vi "executeDefendAreaSkill.vi"(6 "Number of Defenders\nWithout Duelist":i32, 8 "error in (no error)":errorcluster, 9 "Robot in":refnum<class "Robot.lvclass">, 10 "Game":refnum<class "Game.lvclass">, 11 "DefendAreaSkill in":refnum<class "DefendAreaSkill.lvclass">) -> (0 "error out":errorcluster, 2 "Robot out":refnum<class "Robot.lvclass">, 3 "DefendAreaSkill out":refnum<class "DefendAreaSkill.lvclass">)   [LabVIEW 2024, in "DefendAreaSkill.lvclass"]
uses:
  DefendAreaSkill.lvclass
  Game_class/Game.lvclass
  Robot_class/Robot.lvclass
  Utilities_class/Utilities.lvclass
  Team_class/DefensivePlay.ctl
  Team_class/OffensivePlay.ctl
  Game_class/Game.lvclass/Game.ctl
  Parameters_class/Parameters.lvclass/Parameters.ctl
  Team_class/Team.lvclass/Team.ctl
  Robot_class/Robot.lvclass/Robot.ctl
  Game_class/Read Utilities.lvclass.vi
  Game_class/Read FieldRef.vi
  Game_class/Read BallRef.vi
  Robot_class/Write kick_x.vi
  Robot_class/Write kick_z.vi
  Game_class/Read NewParameters.vi
  Game_class/Read OffensiveTeam.vi
  Team_class/Read OffensivePlay.vi
  Game_class/Read Parameters.lvclass.vi
  Game_class/Read DefensiveTeam.vi
  Team_class/Read RobotRef.vi
  Team_class/Read DefensivePlay.vi
  Parameters_class/Read minDistanceToPass.vi
  Parameters_class/Read Enviroment.vi
  Parameters_class/Read MinDistToKick.vi
  Parameters_class/Read ChipKick activated.vi
  Parameters_class/Read ChipKick Force 1.vi
  Parameters_class/Read KickForce.vi
  Parameters_class/Read PassForceMult.vi
  Parameters_class/Read Area.vi
  Robot_class/Write dest_x.vi
  Robot_class/Write dest_y.vi
  Robot_class/Write dest_orientation.vi
  Robot_class/Read orientation.vi
  Ally_class/Ally.lvclass
  C:/Users/ROBOIME2/Documents/SSL ROBOIME/SSL_AI/Team_class/Team.lvclass
  Ball_class/Ball.lvclass
  Parameters_class/Parameters.lvclass
  Field_class/Field.lvclass
  KickToSkill_class/KickToSkill.lvclass
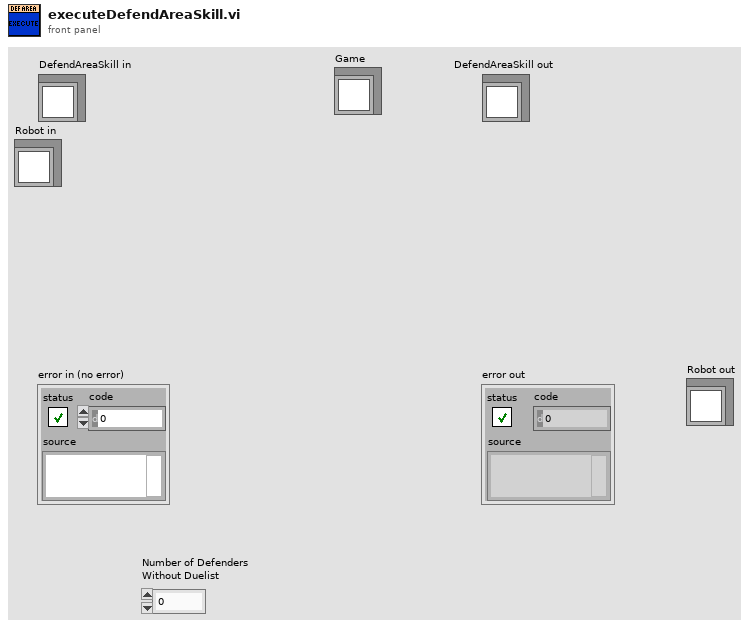
[diagram p1: front panel]
types:
  T1 = typedef "OffensivePlay.ctl" = enum16{"5RobotsPassGamePlay", "5PreparePassGame", "5RobotsKeeperGame", "KeeperPassToStriker", "5RobotsNormalGamePlay", "PrepareKeeperPass", "ACBPass", "ABCPass", "PrepareTriplePass", "TableWithStriker", "TableWith2ndStrikerPlay", "PrepareDoublePass", "PrepareRollToPass", "SimplePass", "PreparePass", "PassToStriker", "BallOutOfField", "PassTo2ndStriker", "StopOffensive", "Prepare Penalty Enemy", "EnemyPossessionAtEnemyField", "EnemyPossesionAtOurField", "TestPlay", "PreparePenaltyAlly", "KickPenaltyAlly", "PrepareKickoffAlly", "PrepareKickoffEnemy", "IndirectEnemy", "DirectEnemy", "PreparePassInGame1", "NormalGame", "DirectKick", "Pass", "Halt", "Timeout", "PassPlay", "PenaltyEnemy"}
  T2 = typedef "DefensivePlay.ctl" = enum16{"NormalDefensiveWithDuelist", "NormalDefensive", "TestPlay", "Halt", "Timeout", "PenaltyEnemy", "PenaltyAlly", "StopDefensive"}
  T3 = typedef "Enviroment.ctl" = enum16{"erForceSimulator", "grSim", "realGame"}
  T4 = typedef "NewParameters.ctl" = cluster{"PenaltyDistance":dbl, "DistanceAttackerToBackBall":dbl, "Division":enum16{"Div B", "Div A"}, "DistanceToAvoidyEnemyRobot":dbl, "BallPlacementDistance":dbl, "DisatanceBehindBallToStealBall":dbl, "MaxDistanceToPositionKickoff":dbl, "BlockEnemyTarget":bool, "MaxStopVAng":dbl, "DistanceMarkerToEnemy":dbl, "IgnoreDribblerContact":bool, "DistanceToBeginEnemyPosession":dbl, "GoToBallWhenEnemyNotMoving":bool, "EnemyDistanceToReduceVelocity":dbl, "TurnOnEnemyDistanceToReduceVelocity":bool, "EnemyDistanceToShootOutBall":dbl, "DefenseKickBall":bool, "MoreKickToGoal? (0-0.3)":dbl, "ChipKickInEnemyField":bool, "ShootOutRobotId":dbl, "FieldLenghtDenominatorInShootOut":dbl, "AdjustPositionInBallPlacement":bool, "PowerGodPass":dbl, "VelocityAbortEnemyPos":dbl, "MaxDistToBeginPass":dbl, "MinDistToBeginPass":dbl, "VelocityInDirects":dbl, "BadDribblerIDs":i32[], "NewKickToDistanceAroundBall":dbl, "PowerAvoidColisionMarker":dbl, "DistanceToAvoidColisionMarker":dbl, "AvoidBallKick":dbl, "DistanceTryKick":dbl, "SuicideKickDIstance":dbl, "AdjustFirstKickDistance":dbl, "AvoidAimLessKick":dbl, "DistanceToAvoidyEnemyShootRobot ":dbl, "NumberOfMarkers":dbl, "PotField":bool, "PIDLateral":bool, "MinDistanceFirstKickX":dbl, "MinDistanceFirstKickY":dbl, "FractionOfDistToTouchGround\nAfterChipKick":dbl, "FractionOfKickxWhen\nComposedWithKickz":dbl, "Style":T5, "MoveInTurnState":bool, "DistFromEnemyToConsider\nMoveInTurnState":dbl, "CascadePID":bool, "TurnAroundParameters":cluster{"Radius":dbl, "Multiplier":dbl, "ChordAngle":dbl}, "SafeDriveVel":dbl, "DistanceToGoToBackBall":dbl, "minDistanceToNotFinish\nEnemyPossession":dbl, "OneTouchShot":cluster{"angleFactor":dbl, "maxAngle":dbl, "Attack":bool, "Defense":bool}, "OpenAngleToGoal":cluster{"minAngle":dbl, "maxAngle":dbl, "minEvaluation":dbl}, "ShotInterception":cluster{"shotSpeed":dbl, "minEnemySpeed":dbl, "maxEnemySpeed":dbl, "minEvaluation":dbl}, "AllyTeamArray":T6[], "maxDefendersNumber":i32, "Zone":cluster{"GuardPositionArray":dbl[][], "ZoneMidField":dbl[], "CenterForwardWidth":dbl}, "MinEvaluationToShoot":dbl, "PassInterception":cluster{"maxPassSpeed":dbl, "minPassSpeed":dbl, "minEnemySpeed":dbl, "chipPassDistance":dbl, "chipPassEvaluation":dbl, "minEvaluation":dbl, "maxEnemySpeed":dbl}, "PassDistance":cluster{"maxDistance":dbl, "minDistance":dbl}, "receiverSpeed":dbl, "maxBallSpeed":dbl, "slackTime":dbl, "Turning radius":dbl, "Turning v_ang":dbl, "AlignError":cluster{"Distance":dbl, "Orientation":dbl, "V_norm(m/s)":dbl, "V_ang (rad/s)":dbl}, "RobotRadius":dbl, "KickerDistance":dbl, "keeper angle  to cover goalpost":dbl, "a_slide":dbl, "a_roll":dbl, "k_switch":dbl}
  T5 = typedef "Style.ctl" = enum16{"Insanity", "Offensive", "Defensive"}
  T6 = typedef "AllyTeam.ctl" = enum16{"Keeper", "Defender", "Attacker"}
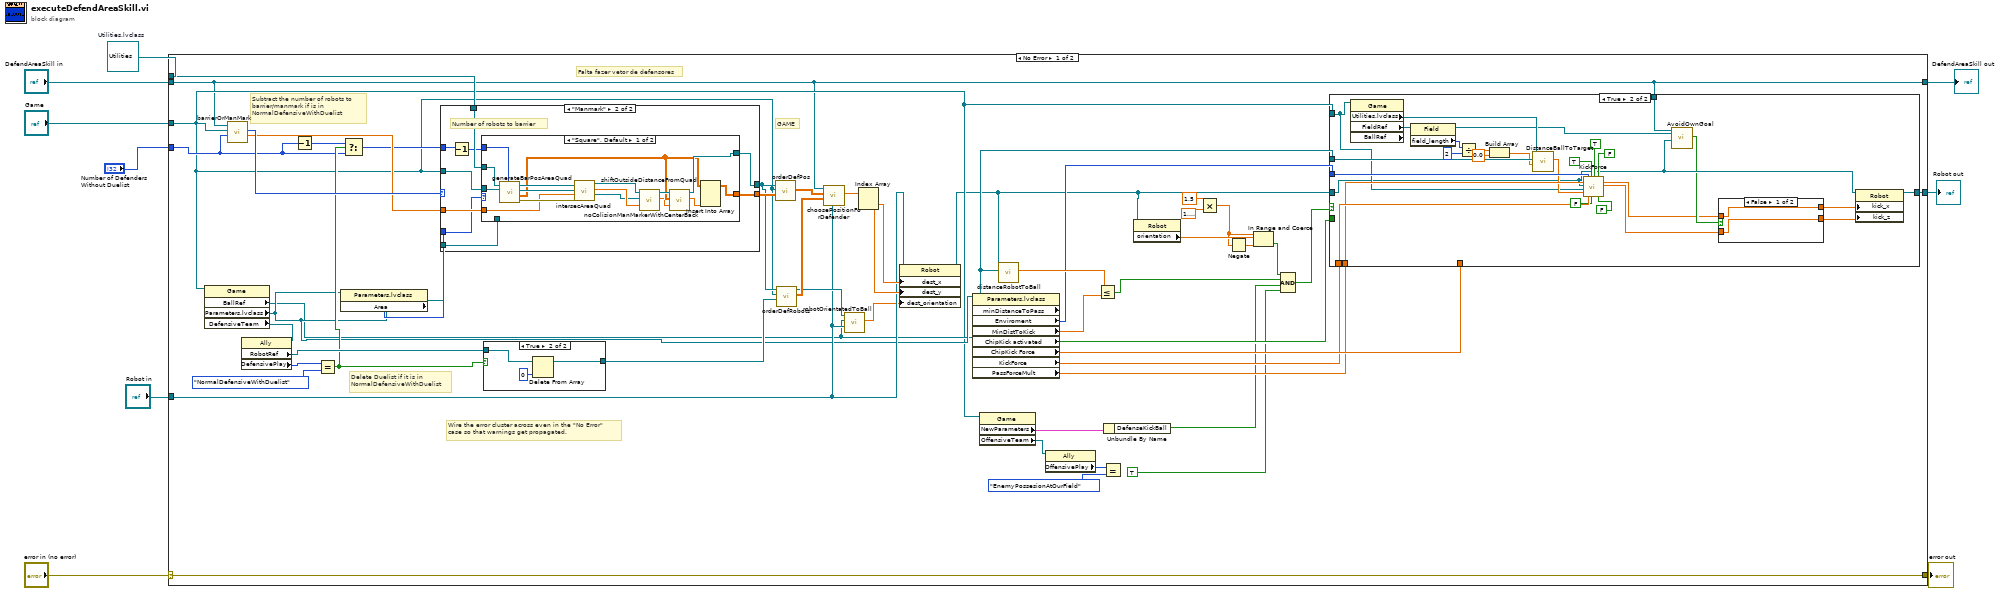
[diagram p0: block diagram]
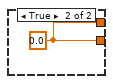
[diagram p3: hidden frame]
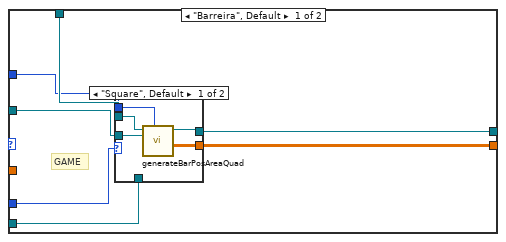
[diagram p5: hidden frame]
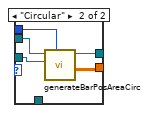
[diagram p6: hidden frame]
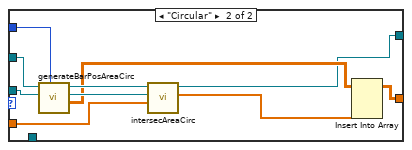
[diagram p7: hidden frame]
diagram:
  w4 = refnum<class "Utilities.lvclass"> refnum  # Utilities.lvclass
  n1 = case shown="No Error" "error in (no error)" {
    selector: "error in (no error)" -> [w60 w150]
    tunnel: [w60 w150] -> w8
    tunnel: [w10 w149] -> w6
    tunnel: "DefendAreaSkill in" -> [w10 w149]
    tunnel: "Game" -> [w24 _]
    tunnel: w4 -> [w58 _]
    tunnel: "Robot in" -> [w48 w148]
    tunnel: [w33 w148] -> w2
    tunnel: "Number of Defenders\nWithout Duelist" -> [w37 _]
    frame No Error {
      # "GAME"
      # "Subtract the number of robots to\nbarrier/manmark if is in\nNormalDefensiveWithDuelist"
      # "Delete Duelist if it is in\nNormalDefensiveWithDuelist"
      # "Falta fazer vetor de defensores"
      # "Wire the error cluster across even in the \"No Error\"\ncase so that warnings get propagated."
      n2 = property class="Game"(reference=w24) -> ("BallRef"=w27:refnum<class "Ball.lvclass">, "Parameters.lvclass"=w35:refnum<class "Parameters.lvclass">, "DefensiveTeam"=w45:refnum<class "Ally.lvclass">)  [unwired: 1 in, 2 out]
      n3 = call "barrierOrManMark.vi"("Number of Defenders\nWithout Duelist"=w37, "Game"=w24, "DefendAreaSkill in"=w10) -> ("Enemy position\nto mark"=w55:dbl[], "Type of Defense Barrier"=w59:enum16{"Barreira", "Manmark"})  [unwired: 5 in, 2 out]
      n4 = property class="Ally"(reference=w45) -> ("RobotRef"=w41:refnum<class "Robot.lvclass">[], "DefensivePlay"=w44:T2)  [unwired: 1 in, 2 out]
      n5 = Decrement(x=w37) -> (x-1=w39:i32)
      n6 = Equal?(x=w44, y=DefensivePlay."NormalDefensiveWithDuelist") -> (x = y?=w40:bool)
      n7 = property class="Parameters.lvclass"(reference=w35) -> ("Area"=w46:enum16{"Circular", "Square"})  [unwired: 1 in, 2 out]
      n8 = Select(t=w39, s=w40, f=w37) -> (s? t:f=w38:i32)
      n9 = case shown="\"Manmark\"" w59 {
        tunnel: w46 -> [w102 w115]
        tunnel: w58 -> [w101 w119]
        tunnel: w35 -> [w100 w121]
        tunnel: w24 -> [w99 w120]
        tunnel: [w98 w117] -> w57
        tunnel: [w97 w116] -> w56
        tunnel: w55 -> [_ w118]
        tunnel: w38 -> [w96 w114]
        frame "Barreira", Default {
          # "GAME"
          n10 = case shown="\"Square\", Default" w102 {
            tunnel: w101 -> [w107 w112]
            tunnel: w100 -> [_ _]
            tunnel: w99 -> [w106 w111]
            tunnel: [w105 w110] -> w97
            tunnel: [w104 w109] -> w98
            tunnel: w96 -> [w103 w108]
            frame "Square", Default {
              n11 = call "generateBarPosAreaQuad.vi"("Number of Defenders\nWithout Duelist"=w103, "Game"=w106, "Utilities in"=w107) -> ("Pos Centers Back"=w104:dbl[][], "Utilities out"=w105:refnum<class "Utilities.lvclass">)  [unwired: 5 in, 2 out]
            }
            frame "Circular" {
              n12 = call "generateBarPosAreaCirc.vi"("Number of Denfenders\nWhithout Duelist"=w108, "Game"=w111, "Utilities in"=w112) -> ("Posição dos Defensores"=w109:dbl[][], "Utilities out"=w110:refnum<class "Utilities.lvclass">)  [unwired: 5 in, 2 out]
            }
          }
        }
        frame "Manmark" {
          # "Number of robots to barrier"
          n13 = Decrement(x=w114) -> (x-1=w113:i32)
          n14 = case shown="\"Square\", Default" w115 {
            tunnel: w119 -> [w137 w147]
            tunnel: w121 -> [_ _]
            tunnel: w120 -> [w136 w146]
            tunnel: w118 -> [w132 w143]
            tunnel: [w131 w140] -> w117
            tunnel: [w125 w139] -> w116
            tunnel: w113 -> [w130 w138]
            frame "Square", Default {
              n15 = call "generateBarPosAreaQuad.vi"("Number of Defenders\nWithout Duelist"=w130, "Game"=w136, "Utilities in"=w137) -> ("error out"=w135:errorcluster, "Pos Centers Back"=w124:dbl[][], "Game out"=w133:refnum<class "Game.lvclass">, "Utilities out"=w134:refnum<class "Utilities.lvclass">)  [unwired: 5 in]
              n16 = call "intersecAreaQuad.vi"("error in (no error)"=w135, "Ball/Enemy\nPosition"=w132, "Game"=w133, "Utilities in"=w134) -> ("Game"=w127:refnum<class "Game.lvclass">, "Pos de Interseção"=w129:dbl[], "Utilities out"=w128:refnum<class "Utilities.lvclass">)  [unwired: 4 in, 1 out]
              n17 = call "shiftOutsideDistanceFromQuad.vi"("Pos de Interseção"=w129, "Game"=w127, "Utilities in"=w128) -> ("Array"=w123:dbl[], "Utilities out"=w126:refnum<class "Utilities.lvclass">)  [unwired: 6 in, 1 out]
              n18 = call "noColisionManMarkerWithCenterBack.vi"("Pos ManMarker 2"=w123, "Pos CenterBacks"=w124, "Utilities in"=w126) -> ("Pos ManMarker"=w122:dbl[], "Utilities out"=w125:refnum<class "Utilities.lvclass">)  [unwired: 6 in, 1 out]
              n19 = Insert Into Array(array=w124, new element=w122) -> (w131:dbl[][])  [unwired: 2 in]
            }
            frame "Circular" {
              n20 = call "generateBarPosAreaCirc.vi"("Number of Denfenders\nWhithout Duelist"=w138, "Game"=w146, "Utilities in"=w147) -> ("Posição dos Defensores"=w142:dbl[][], "Game out"=w144:refnum<class "Game.lvclass">, "Utilities out"=w145:refnum<class "Utilities.lvclass">)  [unwired: 5 in, 1 out]
              n21 = call "intersecAreaCirc.vi"("Ball/Enemy\nPosition"=w143, "Game"=w144, "Utilities in"=w145) -> ("Position"=w141:dbl[], "Utilities out"=w139:refnum<class "Utilities.lvclass">)  [unwired: 6 in, 1 out]
              n22 = Insert Into Array(array=w142, new element=w141) -> (w140:dbl[][])  [unwired: 2 in]
            }
          }
        }
      }
      n23 = case shown="True" w40 {
        tunnel: [w92 w95] -> w42
        tunnel: w41 -> [w92 w94]
        frame False {
        }
        frame True {
          n24 = Delete From Array(array=w94, index=0) -> (array with subset deleted=w95:refnum<class "Robot.lvclass">[])  [unwired: 1 in, 1 out]
        }
      }
      n25 = call "orderDefPos.vi"("Def Positions"=w57, "Game"=w24, "Utilities in"=w56) -> ("Ordered Positions"=w54:dbl[][])  [unwired: 6 in, 2 out]
      n26 = call "orderDefRobots.vi"("Array of Robots"=w42, "Game"=w24, "Utilities in"=w56) -> ("Odered array of robots"=w53:dbl[][], "Utilities out"=w49:refnum<class "Utilities.lvclass">)  [unwired: 6 in, 1 out]
      n27 = call "choosePositionForDefender.vi"("Robot"=w48, "Odered array of robots"=w53, "Ordered Positions To Go"=w54, "DefendAreaSkill in"=w10) -> ("Position"=w52:dbl[])  [unwired: 5 in, 2 out]
      n28 = call "robotOrientatedToBall.vi"("Robot"=w48, "BallRef"=w27, "Utilities in"=w49) -> ("Orientation"=w47:dbl)  [unwired: 6 in, 2 out]
      n29 = Index Array(array=w52) -> (element #1=w51:dbl, element #2=w50:dbl)  [unwired: 2 in]
      n30 = property class="Robot"(reference=w48, "dest_x"=w51, "dest_y"=w50, "dest_orientation"=w47) -> (reference out=w18:refnum<class "Robot.lvclass">)  [unwired: 1 in, 1 out]
      n31 = property class="Parameters.lvclass" props=["minDistanceToPass", "Enviroment", "MinDistToKick", "ChipKick activated", "ChipKick Force", "KickForce", "PassForceMult"](reference=w35) -> ("Enviroment"=w30:T3, "MinDistToKick"=w34:dbl, "ChipKick activated"=w32:bool, "ChipKick Force"=w31:dbl, "KickForce"=w29:dbl, "PassForceMult"=w28:dbl)  [unwired: 1 in, 3 out]
      n32 = property class="Game"(reference=w24) -> ("NewParameters"=w23:T4, "OffensiveTeam"=w21:refnum<class "Ally.lvclass">)  [unwired: 1 in, 2 out]
      n33 = call "distanceRobotToBall.vi"("Robot"=w18, "Ball"=w27) -> ("Distance Robot To Ball"=w36:dbl)  [unwired: 7 in, 2 out]
      n34 = property class="Ally"(reference=w21) -> ("OffensivePlay"=w20:T1)  [unwired: 1 in, 2 out]
      n35 = Less Or Equal?(x=w36, y=w34) -> (x <= y?=w25:bool)
      n36 = Equal?(x=w20, y=OffensivePlay."EnemyPossesionAtOurField") -> ()  [unwired: 1 out]
      n37 = Unbundle By Name(w23) -> ("DefenseKickBall"=w22:bool)
      n38 = property class="Robot"(reference=w18) -> ("orientation"=w17:dbl)  [unwired: 1 in, 2 out]
      n39 = Multiply(x=1.5, y=1.5707963267948966) -> (x*y=w12:dbl)
      n40 = Negate(x=w12) -> (-x=w16:dbl)
      n41 = In Range and Coerce(upper limit=w12, x=w17, lower limit=w16) -> (In Range?=w15:bool)  [unwired: 1 out]
      n42 = Compound Arithmetic op=AND(w15, w25, w22, TRUE ("value")) -> (w26:bool)
      n43 = case shown="True" w26 {
        tunnel: w18 -> [w61 w67]
        tunnel: [w61 w88] -> w33
        tunnel: w32 -> [_ _]
        tunnel: w31 -> [_ _]
        tunnel: w30 -> [_ w87]
        tunnel: w29 -> [_ w85]
        tunnel: w28 -> [_ w84]
        tunnel: w27 -> [_ w83]
        tunnel: w24 -> [_ w73]
        tunnel: w10 -> [_ w69]
        frame False {
        }
        frame True {
          n44 = property class="Game" props=["Utilities.lvclass", "FieldRef", "BallRef"](reference=w73) -> ("Utilities.lvclass"=w75:refnum<class "Utilities.lvclass">, "FieldRef"=w81:refnum<class "Field.lvclass">)  [unwired: 1 in, 3 out]
          n45 = property class="Field"(reference=w81) -> (reference out=w68:refnum<class "Field.lvclass">, "field_length"=w80:i32)  [unwired: 1 in, 1 out]
          n46 = Divide(x=w80, y=2) -> (x/y=w78:dbl)
          n47 = Build Array(w78, 0.0 ("element")) -> (w77:dbl[])
          n48 = call "DistanceBallToTarget.vi"("Target"=w77, "Ball"=w83, "Utilities in"=w75) -> ("Distance Ball To Target"=w82:dbl)  [unwired: 6 in, 2 out]
          n49 = call "KickForce.vi"("force++"=w84, "Robot"=w67, "Game"=w73, "Distance to target"=w82, "Enviroment"=w87, "kickForce"=w85, "chipKick ?"=TRUE, "weakKick?"=FALSE, "shootState?"=TRUE, "use criteria?"=FALSE, "pass?"=FALSE) -> ("kick_x Force out"=w62:dbl, "kick_z Force out"=w63:dbl)  [unwired: 5 in, 2 out]
          n50 = call "AvoidOwnGoal.vi"("DefendAreaSkill in"=w69, "Field"=w68, "Robot"=w67) -> ("Is shooting to our goal?"=w66:bool)  [unwired: 14 in, 2 out]
          n51 = case shown="False" w66 {
            tunnel: [w89 w91] -> w65
            tunnel: [w90 w91] -> w64
            tunnel: w63 -> [w90 _]
            tunnel: w62 -> [w89 _]
            frame False {
            }
            frame True {
              w91 = 0.0
            }
          }
          n52 = property class="Robot"(reference=w67, "kick_x"=w65, "kick_z"=w64) -> (reference out=w88:refnum<class "Robot.lvclass">)  [unwired: 1 in, 1 out]
        }
      }
    }
    frame Error {
    }
  }
  "error out" <- w8
  "DefendAreaSkill out" <- w6
  "Robot out" <- w2
